vi "convert bar to kPa.vi"(7 "P [bar]":dbl[](array[numeric])) -> (8 "P [kPa]":dbl[](array[numeric]))   [LabVIEW 2017, in "util.lvlib"]
uses:
  util.lvlib
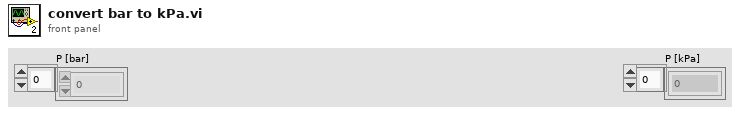
[diagram p1: front panel]
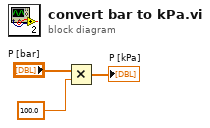
[diagram p0: block diagram]
diagram:
  n1 = Multiply(x="P [bar]", y=100.0) -> (x*y=→"P [kPa]":dbl[])
